vi "test_Create MetaData Channel_error on name collision.vi"(8 "error in (no error)":errorcluster, 11 "TestCase in":refnum<class "Instrument Addon Scripting API Channels Unit Tests.lvclass">) -> (0 "error out":errorcluster, 3 "TestCase out":refnum<class "Instrument Addon Scripting API Channels Unit Tests.lvclass">)   [LabVIEW 2018, in "Instrument Addon Scripting API Channels Unit Tests.lvclass"]
uses:
  Instrument Addon Scripting API Channels Unit Tests.lvclass
  APIs/Scripting API/TypeDefs/Single Channel Type Cast Settings.ctl
  Addon/Addon Shared/Types/Type Cast Type.ctl
  Addon/Addon Shared/Types/Endian.ctl
  APIs/Scripting API/TypeDefs/Single Channel Format Settings.ctl
  Instrument Addon Scripting API Channels Unit Tests.lvclass/Instrument Addon Scripting API Channels Unit Tests.ctl
  <vilib>/NI Veristand/Custom Device Tools/Custom Device Utility Library/NI VeriStand - Search for Item by Name.vi
  APIs/Scripting API/Channels/Create MetaData Channel - Single Channel - Type Cast.vi
  APIs/Scripting API/Channels/Create MetaData Channel - Single Channel - Format.vi
  <vilib>/addons/_JKI Toolkits/VI Tester/TestCase.llb/TestCase.lvclass
  Instrument Addon Scripting API Test Assets/Instrument Addon Scripting API Test Assets.lvclass
  <vilib>/NI Veristand/Custom Device Tools/Custom Device Utility Library/Custom Device Utility Library.lvlib
  Addon/Addon Shared/Instrument Addon Shared.lvlib
  APIs/Scripting API/Instrument Addon Scripting API.lvlib
  C:/Program Files (x86)/National Instruments/LabVIEW 2018/vi.lib/addons/_JKI Toolkits/VI Tester/TestCase.llb/TestCase.lvclass
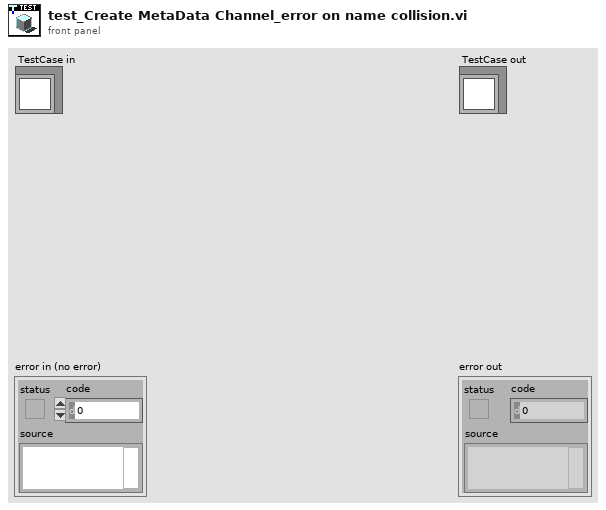
[diagram p1: front panel]
types:
  T1 = typedef "Instrument Addon Scripting API.lvlib/Single Channel Format Settings.ctl" = cluster{"Format String":string, "Default Value":dbl, "Units":string}
  T2 = typedef "Instrument Addon Scripting API.lvlib/Single Channel Type Cast Settings.ctl" = cluster{"Type":T3, "Endian":T4, "Default Value":dbl, "Units":string}
  T3 = typedef "Instrument Addon Shared.lvlib/Type Cast Type.ctl" = enum16{"DBL", "SGL", "U64", "U32", "U16", "U8", "I64", "I32", "I16", "I8"}
  T4 = typedef "Instrument Addon Shared.lvlib/Endian.ctl" = enum16{"Native", "Little", "Big"}
  T5 = typedef "Custom Device API.lvlib/Custom Device Item Ref.ctl" = u64
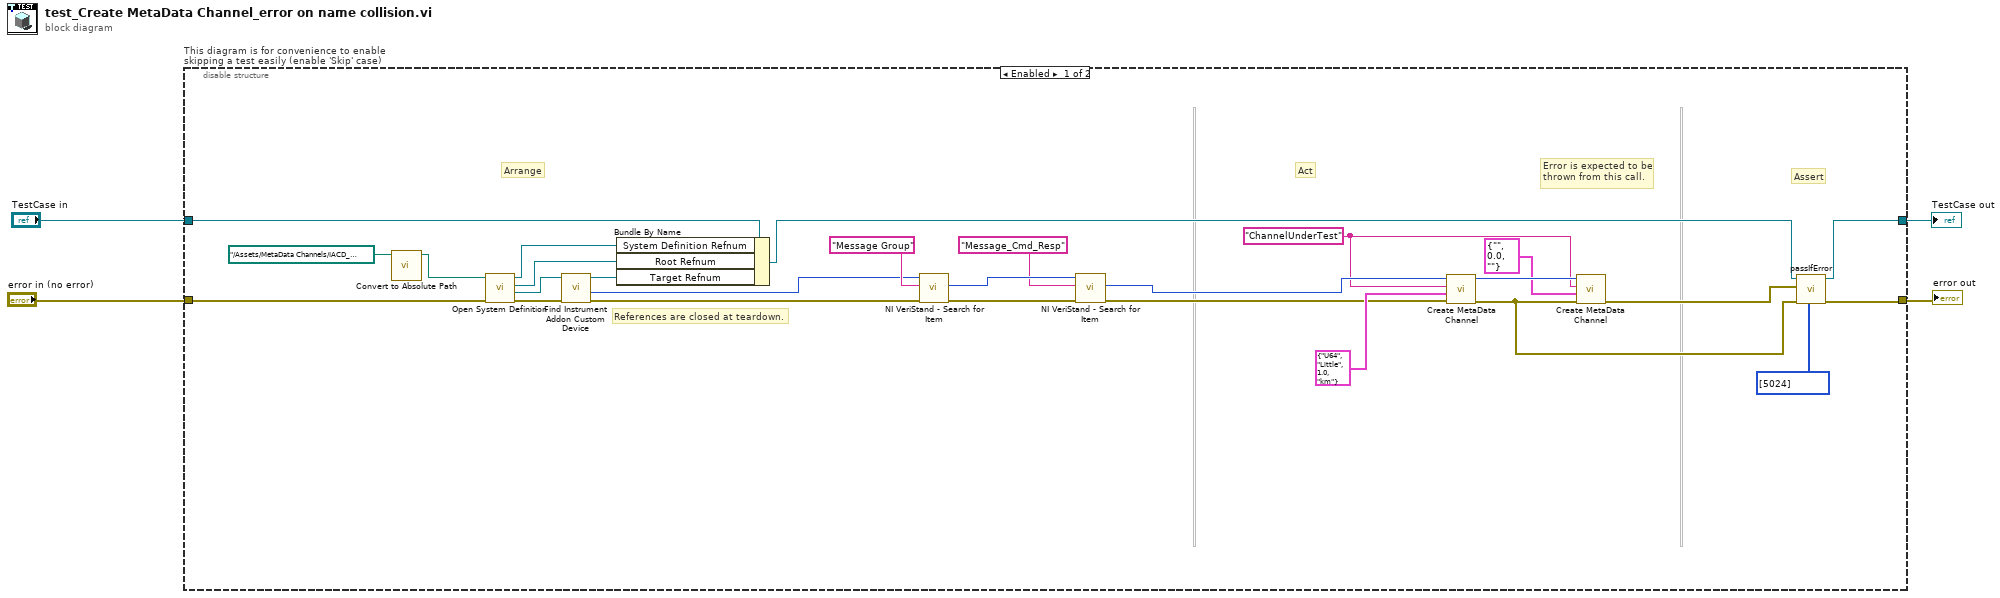
[diagram p0: block diagram]
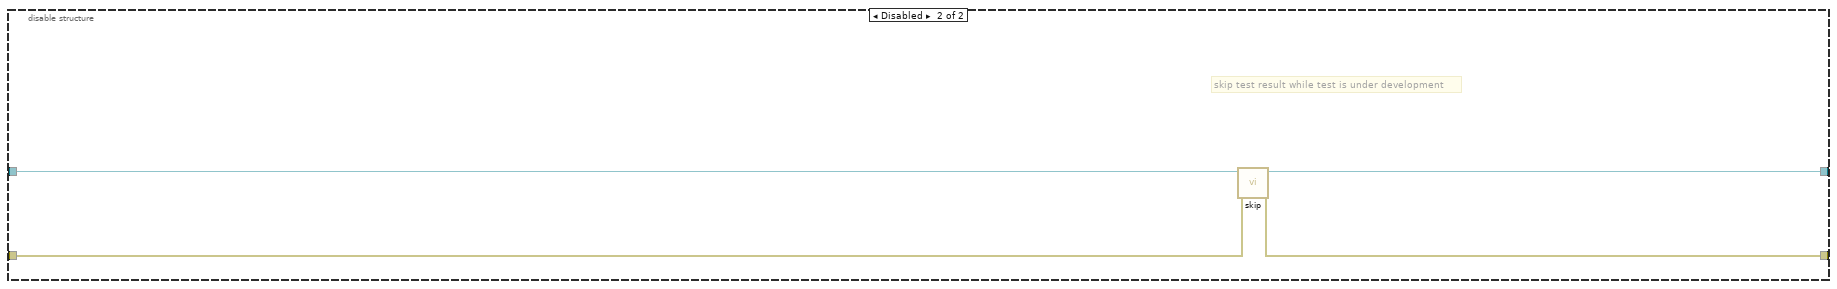
[diagram p2: hidden frame]
diagram:
  n1 = disable-structure "This diagram is for convenience to enable skipping a test easily (enable 'Skip' case)" shown="Enabled" {
    disable-tunnel: "TestCase in" -> [w23 w35]
    disable-tunnel: [w28 w33] -> w1
    disable-tunnel: [w27 w34] -> w3
    disable-tunnel: "error in (no error)" -> [w31 w32]
    frame Enabled {
      w11 = "ChannelUnderTest" ("Name")
      # "Error is expected to be\nthrown from this call."
      # "Assert"
      # "References are closed at teardown."
      # "Act"
      # "Arrange"
      n2 = call "Convert to Absolute Path.vi"("System Definition File"=path "../Assets/MetaData Channels/IACD_channels.nivssdf") -> ("Absolute Path"=w5:path)  [unwired: 10 in]
      n3 = call "Open System Definition.vi"("error in (no error)"=w31, "System Definition File"=w5) -> ("error out"=w29:errorcluster, "Target Refnum"=w30:refnum<k24>, "Root Refnum"=w25:refnum<k24>, "System Definition Refnum"=w24:refnum<k24>)  [unwired: 6 in]
      n4 = call "Find Instrument Addon Custom Device.vi"("error in"=w29, "target in"=w30) -> ("error out"=w18:errorcluster, "NodeID"=w17:u64, "target out"=w26:refnum<k24>)  [unwired: 7 in]
      n5 = Bundle By Name(cluster=w23, "System Definition Refnum"=w24, "Root Refnum"=w25, "Target Refnum"=w26) -> (w13:refnum<class "Instrument Addon Scripting API Channels Unit Tests.lvclass">)
      n6 = call-poly <vilib>:"NI VeriStand - Search for Item.vi"("error in"=w18, "Item Name"="Message Group", "Section Ref in"=w17) -> ("error out"=w19:errorcluster, "Item Ref"=w21:T5)  [unwired: 5 in, 2 out]
      n7 = call-poly <vilib>:"NI VeriStand - Search for Item.vi"("error in"=w19, "Item Name"="Message_Cmd_Resp", "Section Ref in"=w21) -> ("error out"=w14:errorcluster, "Item Ref"=w16:T5)  [unwired: 5 in, 2 out]
      n8 = call-poly "Create MetaData Channel.vi"("Error In"=w14, "Settings"=T2 {"Type"=enum."U64", "Endian"=enum."Little", "Default Value"=1.0, "Units"="km"}, "Name"=w11, "Message Refnum In"=w16) -> ("Error Out"=w7:errorcluster, "Message Refnum Out"=w12:T5)  [unwired: 5 in, 1 out]
      n9 = call-poly "Create MetaData Channel.vi"("Error In"=w7, "Settings"=T1 {"Format String"="", "Default Value"=0.0, "Units"=""}, "Name"=w11, "Message Refnum In"=w12) -> ("Error Out"=w8:errorcluster)  [unwired: 5 in, 2 out]
      n10 = call-dynamic "passIfError.vi"("passing error codes (default = any error code)"=i32[] [5024], "error in (no error)"=w7, "error"=w8, "TestCase in"=w13) -> ("error out"=w27:errorcluster, "TestCase out"=w28:refnum<class "Instrument Addon Scripting API Channels Unit Tests.lvclass">)  [unwired: 6 in]
    }
    frame Disabled {
      # "skip test result while test is under development"
      n11 = call <vilib>:"skip.vi"("error in (no error)"=w32, "TestCase in"=w35) -> ("error out"=w34:errorcluster, "TestCase out"=w33:refnum<class "Instrument Addon Scripting API Channels Unit Tests.lvclass">)  [unwired: 8 in]
    }
  }
  "error out" <- w3
  "TestCase out" <- w1
